vi "testAcquisition.vi"() -> ()   [LabVIEW 2020]
uses:
  HAMAMATSU_DCAMAPI/HAMAMATSU_DCAMAPI.lvclass
  simuCalc Class/simuCalc.lvclass
  Image Acquisition Class/Camera.lvclass
panel:
  out "Frequ [Hz]":dbl
  out "Image":u16[][](graph)
  in  "InClusTiming 2":T1={"Pixelclock"=24, "Exposure"=100.0, "ExposureTimeBase"=1, "Framerate"=14.99615, "TriggerMode"=0} {"TriggerMode" items=["Auto", "Software", "External sequence start ", "External exposure control"]; "ExposureTimeBase" items=["nanoseconds", "microseconds", "milliseconds"]; "Pixelclock" min=1 max=150 step=1 scale=0.05915..150.0; "Framerate" min=0.05915 max=2000.0 step=1.0 scale=0.05915..100.0 scale format="%#.3g"; "Exposure" min=0.001 max=400.0 step=0.001 scale=0.05915..400.0 scale format="%#.3g"}
  in  "ROI":T2={"PosX"=0, "PosY"=0, "Width"=72, "Height"=140} {"PosX" min=0 max=2048 step=1; "Width" min=16 max=2560 step=1; "Height" min=2 max=2160 step=2}
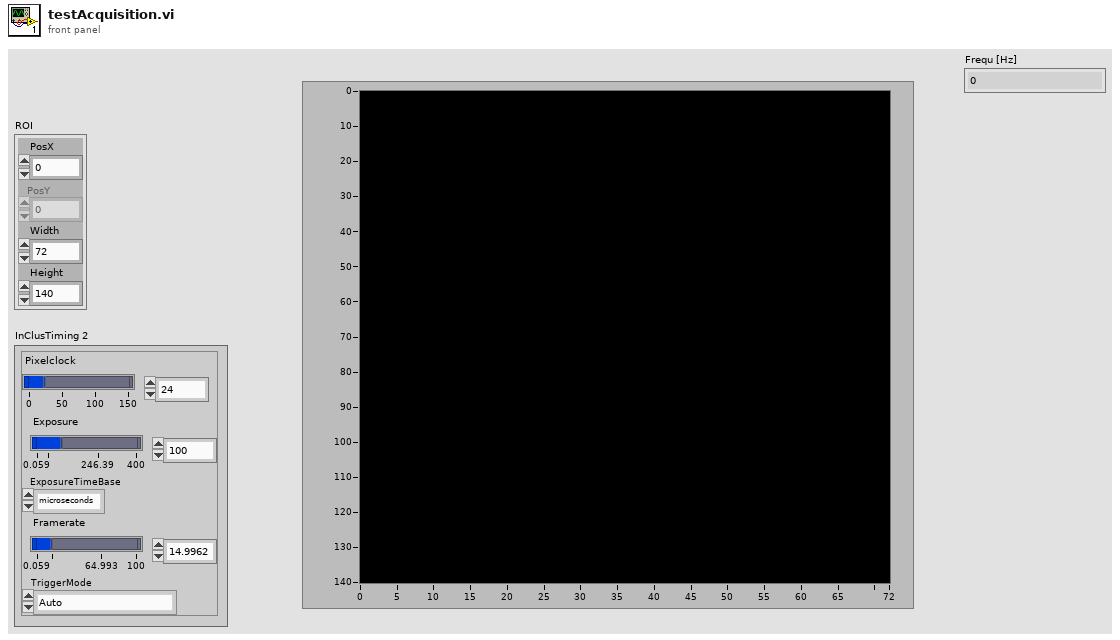
[diagram p1: front panel]
types:
  T1 = cluster{"Pixelclock":i32, "Exposure":dbl, "ExposureTimeBase":u16, "Framerate":dbl, "TriggerMode":u16}
  T2 = cluster{"PosX":i32, "PosY":i32, "Width":i32, "Height":i32}
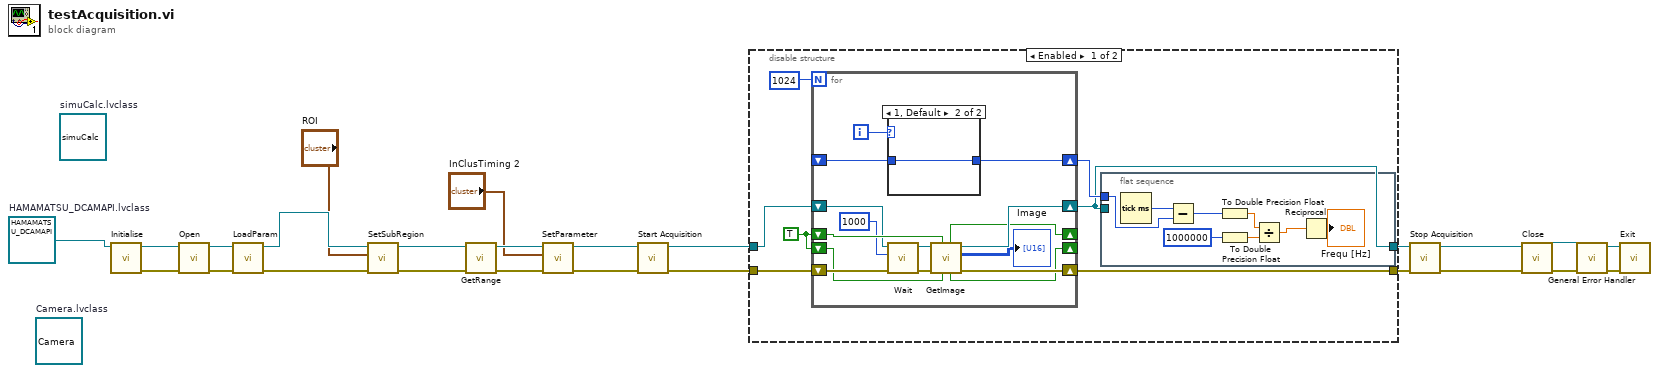
[diagram p0: block diagram]
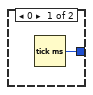
[diagram p2: hidden frame]
diagram:
  w1 = refnum<class "HAMAMATSU_DCAMAPI.lvclass"> refnum  # HAMAMATSU_DCAMAPI.lvclass
  (unwired) refnum<class "Camera.lvclass"> refnum  # Camera.lvclass
  (unwired) refnum<class "simuCalc.lvclass"> refnum  # simuCalc.lvclass
  n1 = call-dynamic "Initialise.vi"("Image Acquisition in"=w1) -> ("error out"=w8:errorcluster, "Image Acquisition out"=w5:refnum<class "HAMAMATSU_DCAMAPI.lvclass">)  [unwired: 9 in]
  n2 = call-dynamic "Open.vi"("error in (no error)"=w8, "HAMAMATSU_DCAMAPI in"=w5) -> ("error out"=w7:errorcluster, "HAMAMATSU_DCAMAPI out"=w6:refnum<class "HAMAMATSU_DCAMAPI.lvclass">)  [unwired: 8 in]
  n3 = call-dynamic "LoadParam.vi"("error in (no error)"=w7, "HAMAMATSU_DCAMAPI in"=w6) -> ("error out"=w24:errorcluster, "HAMAMATSU_DCAMAPI out"=w17:refnum<class "HAMAMATSU_DCAMAPI.lvclass">)  [unwired: 8 in]
  n4 = call-dynamic "SetSubRegion.vi"("error in (no error)"=w24, "ROI"="ROI", "HAMAMATSU_DCAMAPI in"=w17) -> ("error out"=w23:errorcluster, "HAMAMATSU_DCAMAPI out"=w11:refnum<class "HAMAMATSU_DCAMAPI.lvclass">)  [unwired: 7 in]
  n5 = call-dynamic "GetRange.vi"("error in (no error)"=w23, "HAMAMATSU_DCAMAPI in"=w11) -> ("error out"=w22:errorcluster, "HAMAMATSU_DCAMAPI out"=w16:refnum<class "HAMAMATSU_DCAMAPI.lvclass">)  [unwired: 8 in]
  n6 = call-dynamic "SetParameter.vi"("error in (no error)"=w22, "InClusTiming"="InClusTiming 2", "HAMAMATSU_DCAMAPI in"=w16) -> ("error out"=w21:errorcluster, "HAMAMATSU_DCAMAPI out"=w15:refnum<class "HAMAMATSU_DCAMAPI.lvclass">)  [unwired: 7 in]
  n7 = call-dynamic "Start Acquisition.vi"("error in (no error)"=w21, "Image Acquisition in"=w15) -> ("error out"=w3:errorcluster, "Image Acquisition out"=w2:refnum<class "HAMAMATSU_DCAMAPI.lvclass">)  [unwired: 8 in]
  n8 = disable-structure shown="Enabled" {
    disable-tunnel: w3 -> [w31 w58]
    disable-tunnel: [w30 w58] -> w20
    disable-tunnel: w2 -> [w29 w57]
    disable-tunnel: [w25 w57] -> w14
    frame Enabled {
      w28 = TRUE ("bUseBuffer0")
      n9 = for {
        N: 1024 -> [_]
        shift-right: [w53] -> w30
        shift-left: w31 -> [w54]
        shift-right: [w52] -> w25
        shift-left: w29 -> [w45]
        shift-right: [w49] -> _
        shift-left: w28 -> [w48]
        shift-right: [w50] -> _
        shift-left: w28 -> [w51]
        shift-right: [w41] -> w26
        shift-left: _ -> [w40]
        i -> [w42]
        n10 = case shown="1, Default" w42 {
          tunnel: [w55 w56] -> w41
          tunnel: w40 -> [_ w56]
          frame 0 {
            n11 = Tick Count (ms)() -> (millisecond timer value=w55:u32)
          }
          frame 1, Default {
          }
        }
        n12 = call-dynamic "Wait.vi"("error in (no error)"=w54, "Timeout"=1000, "HAMAMATSU_DCAMAPI in"=w45) -> ("error out"=w46:errorcluster, "HAMAMATSU_DCAMAPI out"=w44:refnum<class "HAMAMATSU_DCAMAPI.lvclass">)  [unwired: 7 in]
        n13 = call-dynamic "GetImage.vi"("bUseBuffer1"=w51, "bUseBuffer0"=w48, "error in (no error)"=w46, "Image Acquisition in"=w44) -> ("error out"=w53:errorcluster, "Image Reference"=→"Image":u16[][], "Image Acquisition out"=w52:refnum<class "HAMAMATSU_DCAMAPI.lvclass">, "bUseBuffer1"=w50:bool, "bUseBuffer0"=w49:bool)  [unwired: 2 in, 1 out]
      }
      n14 = flat-sequence {
        tunnel: w26 -> [w38]
        tunnel: w25 -> [_]
        frame #0 {
          n15 = Tick Count (ms)() -> (millisecond timer value=w39:u32)
          n16 = Subtract(x=w39, y=w38) -> (x-y=w37:u32)
          n17 = To Double Precision Float(number=w37) -> (double precision float=w34:dbl)
          n18 = To Double Precision Float(number=u32 1000000 ("y")) -> (double precision float=w33:dbl)
          n19 = Divide(x=w34, y=w33) -> (x/y=w36:dbl)
          n20 = Reciprocal(x=w36) -> (1/x=→"Frequ [Hz]":dbl)
        }
      }
    }
    frame Disabled {
    }
  }
  n21 = call-dynamic "Stop Acquisition.vi"("error in (no error)"=w20, "HAMAMATSU_DCAMAPI in"=w14) -> ("error out"=w19:errorcluster, "HAMAMATSU_DCAMAPI out"=w13:refnum<class "HAMAMATSU_DCAMAPI.lvclass">)  [unwired: 8 in]
  n22 = call-dynamic "Close.vi"("error in (no error)"=w19, "HAMAMATSU_DCAMAPI in"=w13) -> ("error out"=w18:errorcluster, "HAMAMATSU_DCAMAPI out"=w12:refnum<class "HAMAMATSU_DCAMAPI.lvclass">)  [unwired: 8 in]
  n23 = call <vilib>:"General Error Handler.vi"("error in (no error)"=w18) -> ("error out"=w4:errorcluster)  [unwired: 10 in, 4 out]
  n24 = call-dynamic "Exit.vi"("error in (no error)"=w4, "Image Acquisition in"=w12) -> ()  [unwired: 8 in, 2 out]
